vi "STM32_Labview.vi"() -> ()   [LabVIEW 2020]
uses:
  <vilib>/Utility/file.llb/Write Delimited Spreadsheet (string).vi
  <vilib>/Instr/_visa.llb/VISA Configure Serial Port (Instr).vi
panel:
  out "Iteração Atual":i32
  out "Total Iterações":i8
  in  "Incremento":dbl
  in  "Valor Final":dbl
  in  "Valor Inicial":dbl
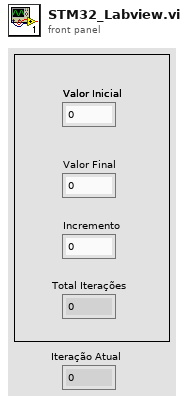
[diagram p1: front panel]
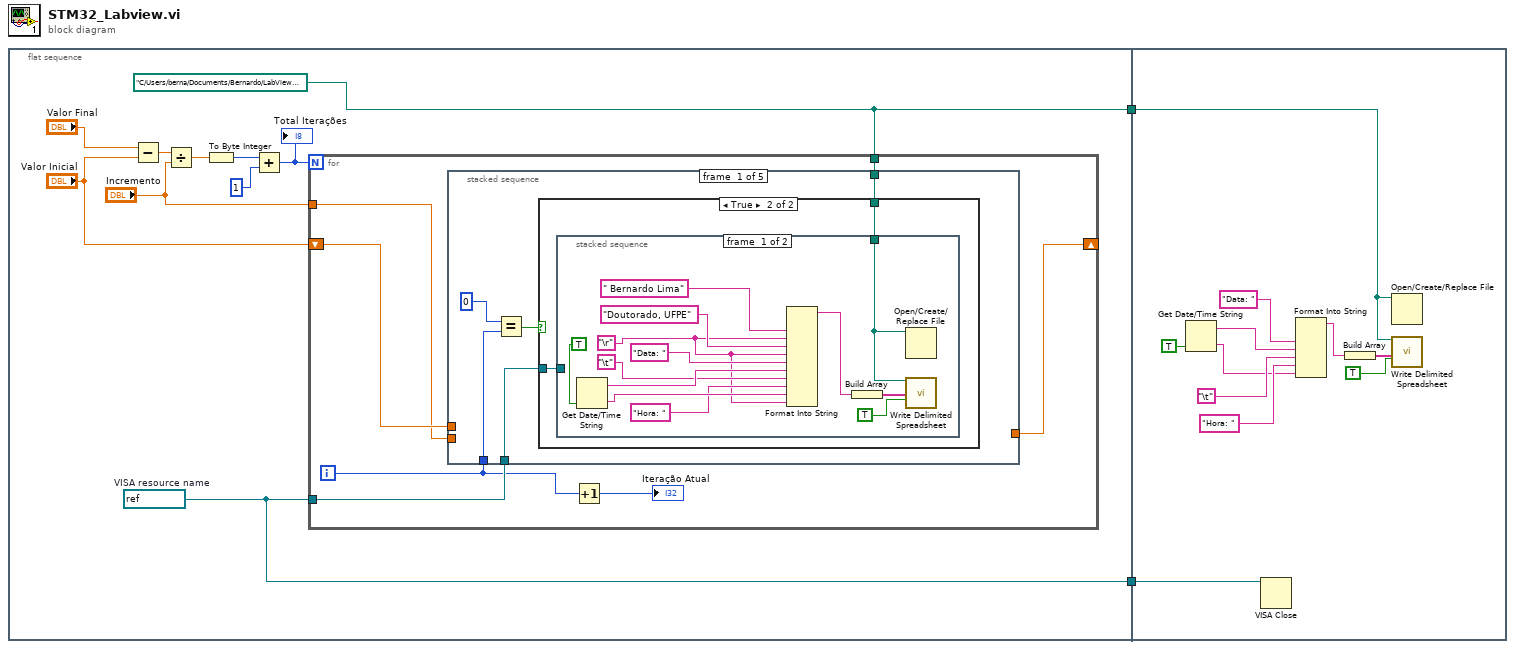
[diagram p0: block diagram]
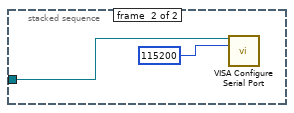
[diagram p3: hidden frame]
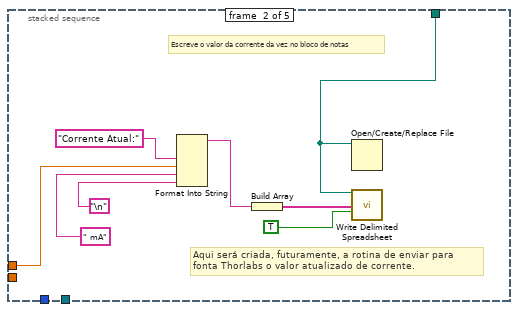
[diagram p4: hidden frame]
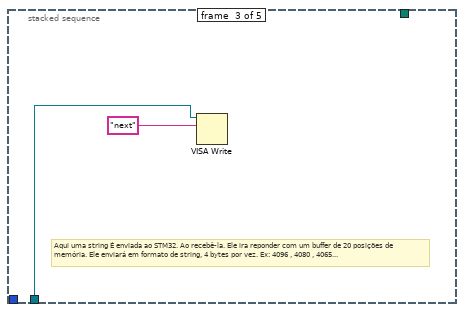
[diagram p5: hidden frame]
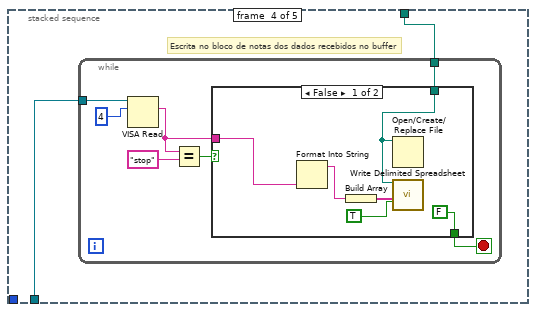
[diagram p6: hidden frame]
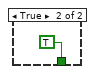
[diagram p7: hidden frame]
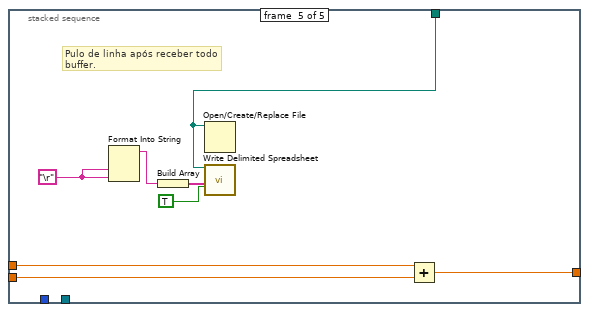
[diagram p8: hidden frame]
diagram:
  n1 = flat-sequence {
    tunnel: [w7] -> w2
    tunnel: [w3] -> w1
    tunnel: w2 -> [w86]
    tunnel: w1 -> [w76]
    frame #0 {
      w3 = path "C:/Users/berna/Documents/Bernardo/LabView Projetos/STM32_LabView/texto.txt" ("file path (use dialog)")
      w7 = refnum<visa-resource-name> "COM3"  # VISA resource name
      n2 = Subtract(x="Valor Final", y="Valor Inicial") -> (x-y=w11:dbl)
      n3 = Divide(x=w11, y="Incremento") -> (x/y=w10:dbl)
      n4 = To Byte Integer(number=w10) -> (8bit integer=w5:i8)
      n5 = Add(x=w5, y=i8 1) -> (x+y=w4:i8)
      "Total Iterações" <- w4
      n6 = for {
        N: w4 -> [_]
        shift-right: [w17] -> _
        shift-left: "Valor Inicial" -> [w19]
        tunnel: w7 -> [w16]
        tunnel: "Incremento" -> [w18]
        tunnel: w3 -> [w15]
        i -> [w13]
        n7 = stacked-sequence {
          tunnel: w19 -> [_ w45 _ _ w70]
          tunnel: w13 -> [w24 _ _ _ _]
          tunnel: w16 -> [w21 _ w50 w53 _]
          tunnel: w18 -> [_ _ _ _ w71]
          tunnel: [_ _ _ _ w69] -> w17
          tunnel: w15 -> [w20 w42 _ w52 w68]
          frame #0 {
            n8 = Equal?(x=0, y=w24) -> (x = y?=w22:bool)
            n9 = case shown="True" w22 {
              tunnel: w21 -> [_ w26]
              tunnel: w20 -> [_ w25]
              frame False {
              }
              frame True {
                n10 = stacked-sequence {
                  tunnel: w26 -> [_ w41]
                  tunnel: w25 -> [w27 _]
                  frame #0 {
                    w29 = "\r"
                    n11 = Get Date/Time String(want seconds? (F)=TRUE) -> (date string=w33:string, time string=w31:string)  [unwired: 2 in]
                    n12 = Format Into String(" Bernardo Lima", w29, "Doutorado, UFPE", w29, "Data: ", w33, "\t", "Hora: ", w31, w29) -> (resulting string=w38:string)  [unwired: 3 in, 1 out]
                    n13 = Build Array(w38) -> (w37:string[])
                    n14 = Open/Create/Replace File(file path (use dialog)=w27) -> ()  [unwired: 5 in, 3 out]
                    n15 = call-poly <vilib>:"Write Delimited Spreadsheet.vi"("file path (dialog if empty)"=w27, "1D data"=w37, "append to file? (new file:F)"=TRUE) -> ()  [unwired: 11 in, 2 out]
                  }
                  frame #1 {
                    n16 = call-poly "VISA Configure Serial Port"("VISA resource name"=w41, "baud rate (9600)"=u32 115200) -> ()  [unwired: 12 in, 2 out]
                  }
                }
              }
            }
          }
          frame #1 {
            # "Escreve o valor da corrente da vez no bloco de notas"
            # "Aqui será criada, futuramente, a rotina de enviar para fonta Thorlabs o valor atualizado de corrente."
            n17 = Format Into String("Corrente Atual:", w45, " mA", "\n") -> (resulting string=w48:string)  [unwired: 3 in, 1 out]
            n18 = Build Array(w48) -> (w47:string[])
            n19 = Open/Create/Replace File(file path (use dialog)=w42) -> ()  [unwired: 5 in, 3 out]
            n20 = call-poly <vilib>:"Write Delimited Spreadsheet.vi"("file path (dialog if empty)"=w42, "1D data"=w47, "append to file? (new file:F)"=TRUE) -> ()  [unwired: 11 in, 2 out]
          }
          frame #2 {
            # "Aqui uma string É enviada ao STM32. Ao recebê-la. Ele ira reponder com um buffer de 20 posições de memória. Ele enviará em formato de string, 4 bytes por vez. Ex: 4096 , 4080 , 4065..."
            n21 = VISA Write(VISA resource name=w50, write buffer="next") -> ()  [unwired: 1 in, 3 out]
          }
          frame #3 {
            # "Escrita no bloco de notas dos dados recebidos no buffer"
            n22 = while {
              tunnel: w53 -> [w60]
              tunnel: w52 -> [w54]
              stop <- w56 stop-if-true
              n23 = VISA Read(VISA resource name=w60, byte count=u32 4) -> (read buffer=w55:string)  [unwired: 1 in, 3 out]
              n24 = Equal?(x=w55, y="stop") -> (x = y?=w57:bool)
              n25 = case shown="False" w57 {
                tunnel: [FALSE TRUE] -> w56
                tunnel: w55 -> [w62 _]
                tunnel: w54 -> [w61 _]
                frame False {
                  n26 = Format Into String(w62) -> (resulting string=w65:string)  [unwired: 3 in, 1 out]
                  n27 = Build Array(w65) -> (w64:string[])
                  n28 = Open/Create/Replace File(file path (use dialog)=w61) -> ()  [unwired: 5 in, 3 out]
                  n29 = call-poly <vilib>:"Write Delimited Spreadsheet.vi"("file path (dialog if empty)"=w61, "1D data"=w64, "append to file? (new file:F)"=TRUE) -> ()  [unwired: 11 in, 2 out]
                }
                frame True {
                }
              }
            }
          }
          frame #4 {
            w72 = "\r"
            # "Pulo de linha após receber todo buffer."
            n30 = Format Into String(w72, w72) -> (resulting string=w75:string)  [unwired: 3 in, 1 out]
            n31 = Build Array(w75) -> (w74:string[])
            n32 = Open/Create/Replace File(file path (use dialog)=w68) -> ()  [unwired: 5 in, 3 out]
            n33 = call-poly <vilib>:"Write Delimited Spreadsheet.vi"("file path (dialog if empty)"=w68, "1D data"=w74, "append to file? (new file:F)"=TRUE) -> ()  [unwired: 11 in, 2 out]
            n34 = Add(x=w70, y=w71) -> (x+y=w69:dbl)
          }
        }
        n35 = Increment(x=w13) -> (x+1=→"Iteração Atual":i32)
      }
    }
    frame #1 {
      n36 = Get Date/Time String(want seconds? (F)=TRUE) -> (date string=w79:string, time string=w77:string)  [unwired: 2 in]
      n37 = VISA Close(VISA resource name=w86) -> ()  [unwired: 1 in, 1 out]
      n38 = Format Into String("Data: ", w79, "\t", "Hora: ", w77) -> (resulting string=w85:string)  [unwired: 3 in, 1 out]
      n39 = Build Array(w85) -> (w84:string[])
      n40 = Open/Create/Replace File(file path (use dialog)=w76) -> ()  [unwired: 5 in, 3 out]
      n41 = call-poly <vilib>:"Write Delimited Spreadsheet.vi"("file path (dialog if empty)"=w76, "1D data"=w84, "append to file? (new file:F)"=TRUE) -> ()  [unwired: 11 in, 2 out]
    }
  }
